vi "Async.Engine.Write Data to HW.vi"(8 "error in":errorcluster, 11 "VS Plugin Inline Async API in":refnum<class "VS Plugin Inline Async API.lvclass">=refnum) -> (0 "error out":errorcluster, 3 "VS Plugin Inline Async API out":refnum<class "VS Plugin Inline Async API.lvclass">)   [LabVIEW 2023, in "VS Plugin Inline Async API.lvlib" / "VS Plugin Inline Async API.lvclass"]
uses:
  VS Plugin Inline Async API.lvclass
  VS Plugin Inline Async API.lvclass/VS Plugin Inline Async API.ctl
  _Plugin Data Access Engine/Plugin Data Access Engine/Plugin Data Access Engine.lvclass
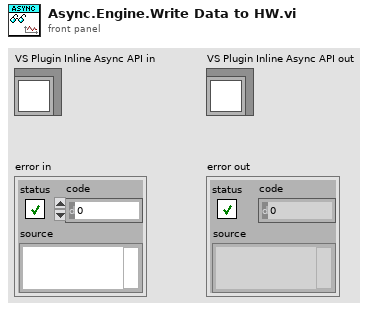
[diagram p1: front panel]
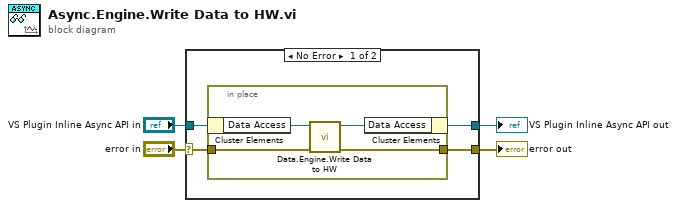
[diagram p0: block diagram]
diagram:
  n1 = case shown="No Error" "error in" {
    selector: "error in" -> [w6 w14]
    tunnel: [w5 w14] -> w3
    tunnel: [w7 w13] -> w1
    tunnel: "VS Plugin Inline Async API in" -> [w8 w13]
    frame No Error {
      n2 = in-place {
        in-place-border: w6 -> [w12]
        in-place-border: [w9] -> w5
        n3 = in-place-cluster #1(w8) -> ("Data Access"=w11:refnum<class "Plugin Data Access Engine.lvclass">)
        n4 = call "Data.Engine.Write Data to HW.vi"("error in"=w12, "Data Access API in"=w11) -> ("error out"=w9:errorcluster, "Data Access API out"=w10:refnum<class "Plugin Data Access Engine.lvclass">)  [unwired: 8 in]
        n5 = in-place-cluster #1("Data Access"=w10) -> (w7:refnum<class "VS Plugin Inline Async API.lvclass">)
      }
    }
    frame Error {
    }
  }
  "error out" <- w3
  "VS Plugin Inline Async API out" <- w1
